vi "InitializeObstacle.vi"(10 "Enclose obstacle? (T)":bool=TRUE, 11 "Input List of UTM locations to be arranged into segments":T1[](array[typedef]) {"North" format="%#_10f"; "East" format="%#_8f"}) -> (3 "Obstacle.lvclass":refnum<class "Obstacle.lvclass">)   [LabVIEW 2013, in "Obstacle.lvclass"]
doc: "Gets an input of a list of points, outputs an obstacle. Final segment is the last and first segments. This traces the given UTM coordinates and creates line segments from each to the next, wrapping around from the last to the first. Could potentially create an obstacle like an enclosed island from this.\n\nEdited Eric Schneider, August 2014"
uses:
  Obstacle.lvclass
  Data/TypeDefs/UTM Location.ctl
  Obstacle.lvclass/Obstacle.ctl
panel:
  in  "Point Cluster":cluster{"Point 1":T1, "Point 0":T1} {"Point 0"."North" format="%#_10f"; "Point 0"."East" format="%#_8f"; "Point 1"."North" format="%#_10f"; "Point 1"."East" format="%#_8f"}
  in  "Obstacle.lvclass":refnum<class "Obstacle.lvclass">
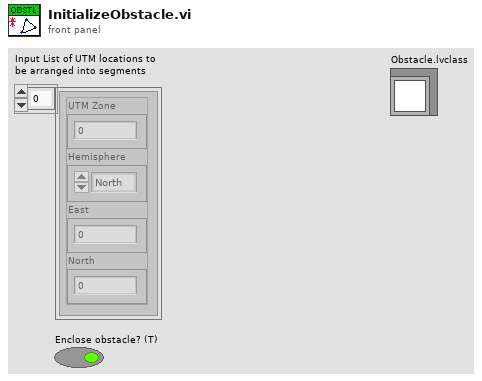
[diagram p1: front panel]
types:
  T1 = typedef "UTM Location.ctl" = cluster{"UTM Zone":dbl, "Hemisphere":enum16{"North", "South"}, "East":dbl, "North":dbl}
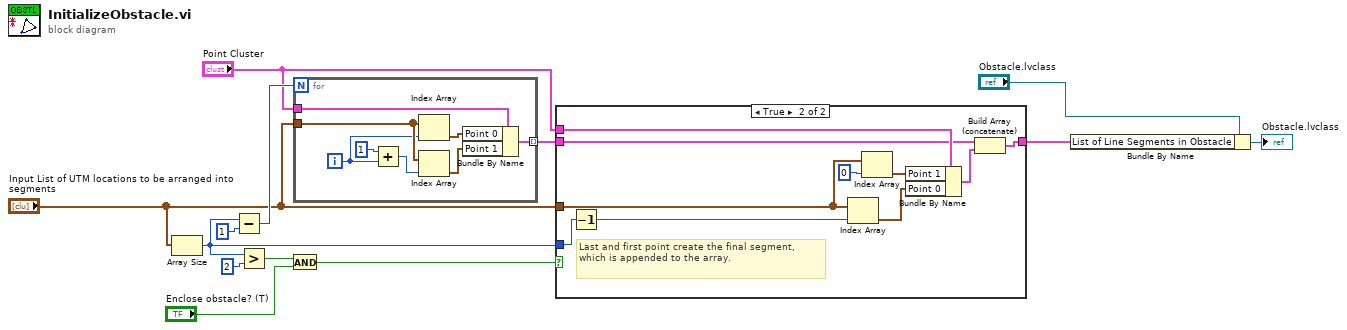
[diagram p0: block diagram]
diagram:
  n1 = Array Size(array="Input List of UTM locations to be arranged into segments") -> (size(s)=w5:i32)
  n2 = Subtract(x=w5, y=1) -> (x-y=w13:i32)
  n3 = Greater?(x=w5, y=2) -> (0:w3:bool)
  n4 = And(x=w3, y="Enclose obstacle? (T)") -> (x .and. y?=w1:bool)
  n5 = for {
    N: w13 -> [_]
    tunnel: "Input List of UTM locations to be arranged into segments" -> [w21]
    tunnel: [w15] -> w7 mode=indexing
    tunnel: "Point Cluster" -> [w14]
    i -> [w18]
    n6 = Add(x=1, y=w18) -> (x+y=w20:i32)
    n7 = Index Array(array=w21, index=w18) -> (element=w17:T1)
    n8 = Index Array(array=w21, index=w20) -> (element=w16:T1)
    n9 = Bundle By Name(cluster=w14, "Point 0"=w17, "Point 1"=w16) -> (w15:cluster{"Point 1":T1, "Point 0":T1})
  }
  n10 = case shown="True" w1 {
    tunnel: w5 -> [_ w28]
    tunnel: "Point Cluster" -> [_ w27]
    tunnel: "Input List of UTM locations to be arranged into segments" -> [_ w26]
    tunnel: w7 -> [w22 w25]
    tunnel: [w22 w23] -> w6
    frame False {
    }
    frame True {
      # "Last and first point create the final segment, which is appended to the array."
      n11 = Decrement(x=w28) -> (x-1=w32:i32)
      n12 = Index Array(array=w26, index=w32) -> (element=w31:T1)
      n13 = Index Array(array=w26, index=0) -> (element=w30:T1)
      n14 = Bundle By Name(cluster=w27, "Point 1"=w30, "Point 0"=w31) -> (w24:cluster{"Point 1":T1, "Point 0":T1})
      n15 = Build Array (concatenate)(w25, w24) -> (w23:cluster{"Point 1":T1, "Point 0":T1}[])
    }
  }
  n16 = Bundle By Name(cluster="Obstacle.lvclass", "List of Line Segments in Obstacle"=w6) -> (→"Obstacle.lvclass":refnum<class "Obstacle.lvclass">)
